vi "Configure Automask.vi"(6 "Horizontal Tolerance":dbl, 7 "Vertical Tolerance":dbl, 8 "error in (no error)":errorcluster, 9 "Units (0: Volts/Time)":i32(ring) items=["Volts/Time", "Divisions"], 10 "Channel (1: Channel 1)":i32(ring)=1 items=["Channel 1"=1, "Channel 2"=2, "Channel 3"=3, "Channel 4"=4], 11 "VISA resource name":refnum<visa-resource-name>) -> (0 "error out":errorcluster, 3 "VISA resource name out":refnum<visa-resource-name>)   [LabVIEW 2020, in "Agilent 90000 Series.lvlib"]
doc: "Configures the automask parameters."
uses:
  Agilent 90000 Series.lvlib
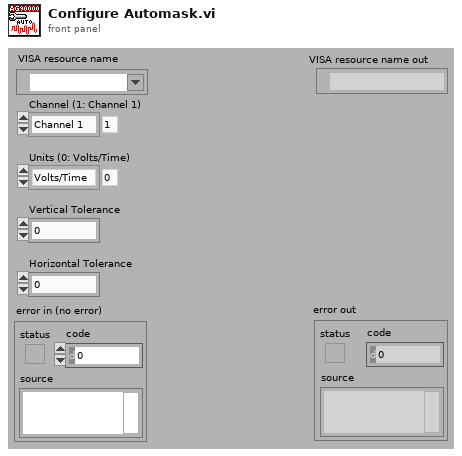
[diagram p1: front panel]
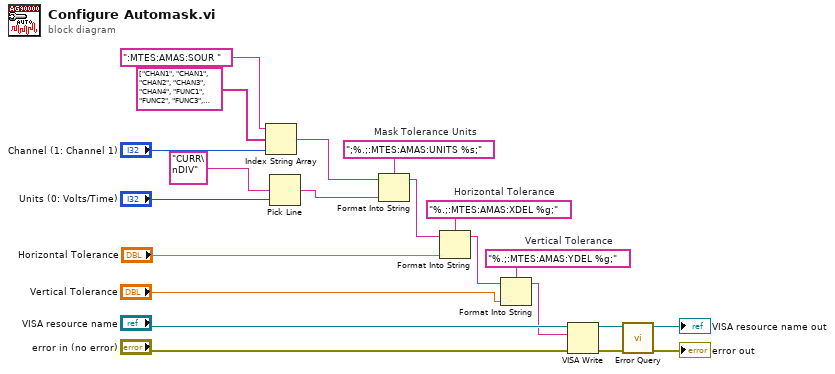
[diagram p0: block diagram]
diagram:
  w5 = "%.;:MTES:AMAS:YDEL %g;"  # Vertical Tolerance
  w8 = "%.;:MTES:AMAS:XDEL %g;"  # Horizontal Tolerance
  w13 = ";%.;:MTES:AMAS:UNITS %s;"  # Mask Tolerance Units
  n1 = Index String Array(1:"Channel (1: Channel 1)", 2:string[] ["CHAN1", "CHAN1", "CHAN2", "CHAN3", "CHAN4", "FUNC1", "FUNC2", "FUNC3", "FUNC4", "WMEM1", "WMEM2", "WMEM3", "WMEM4"] ("subarray 2"), 3:":MTES:AMAS:SOUR " ("string (\"\")")) -> (0:w10:string)
  n2 = Pick Line(multi-line string="CURR\nDIV", line index="Units (0: Volts/Time)") -> (output string=w11:string)  [unwired: 1 out]
  n3 = Format Into String(format string=w13, initial string=w10, w11) -> (resulting string=w2:string)  [unwired: 1 in, 1 out]
  n4 = Format Into String(format string=w8, initial string=w2, "Horizontal Tolerance") -> (resulting string=w3:string)  [unwired: 1 in, 1 out]
  n5 = Format Into String(format string=w5, initial string=w3, "Vertical Tolerance") -> (resulting string=w4:string)  [unwired: 1 in, 1 out]
  n6 = VISA Write(VISA resource name="VISA resource name", write buffer=w4, error in (no error)="error in (no error)") -> (VISA resource name out=w19:refnum<visa-resource-name>, error out=w18:errorcluster)  [unwired: 1 out]
  n7 = call "Error Query.vi"("error in (no error)"=w18, "VISA resource name"=w19) -> ("error out"=→"error out":errorcluster, "VISA resource name out"=→"VISA resource name out":refnum<visa-resource-name>)  [unwired: 8 out]
